vi "SeCrTs-Data queue.vi"(3 "error in":errorcluster) -> (7 "Data FIFO Ref":T1, 10 "error out":errorcluster)   [LabVIEW 2022 SP3]
uses:
  RT Controls/SeCrTs-Data FIFO.ctl
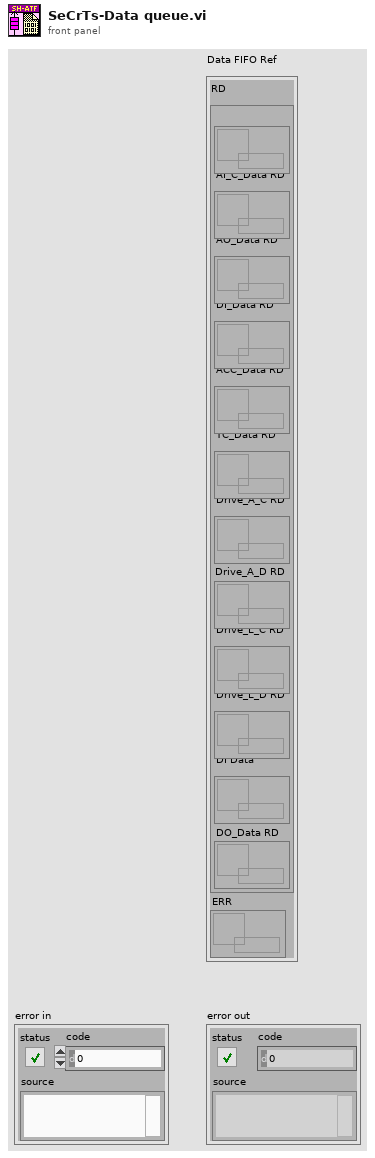
[diagram p1: front panel]
types:
  T1 = typedef "SeCrTs-Data FIFO.ctl" = cluster{"RD":cluster{"AI_V_Data RD":refnum<queue>, "AI_C_Data RD":refnum<queue>, "AO_Data RD":refnum<queue>, "DI_Data RD":refnum<queue>, "ACC_Data RD":refnum<queue>, "TC_Data RD":refnum<queue>, "Drive_A_C RD":refnum<queue>, "Drive_A_D RD":refnum<queue>, "Drive_L_C RD":refnum<queue>, "Drive_L_D RD":refnum<queue>, "DI Data":refnum<queue>, "DO_Data RD":refnum<queue>}, "ERR":refnum<queue>}
  T2 = cluster{"Error Code":string, "Error Source":string}
  T3 = cluster{"AI_V_Data RD":refnum<queue>, "AI_C_Data RD":refnum<queue>, "AO_Data RD":refnum<queue>, "DI_Data RD":refnum<queue>, "ACC_Data RD":refnum<queue>, "TC_Data RD":refnum<queue>, "Drive_A_C RD":refnum<queue>, "Drive_A_D RD":refnum<queue>, "Drive_L_C RD":refnum<queue>, "Drive_L_D RD":refnum<queue>, "DI Data":refnum<queue>, "DO_Data RD":refnum<queue>}
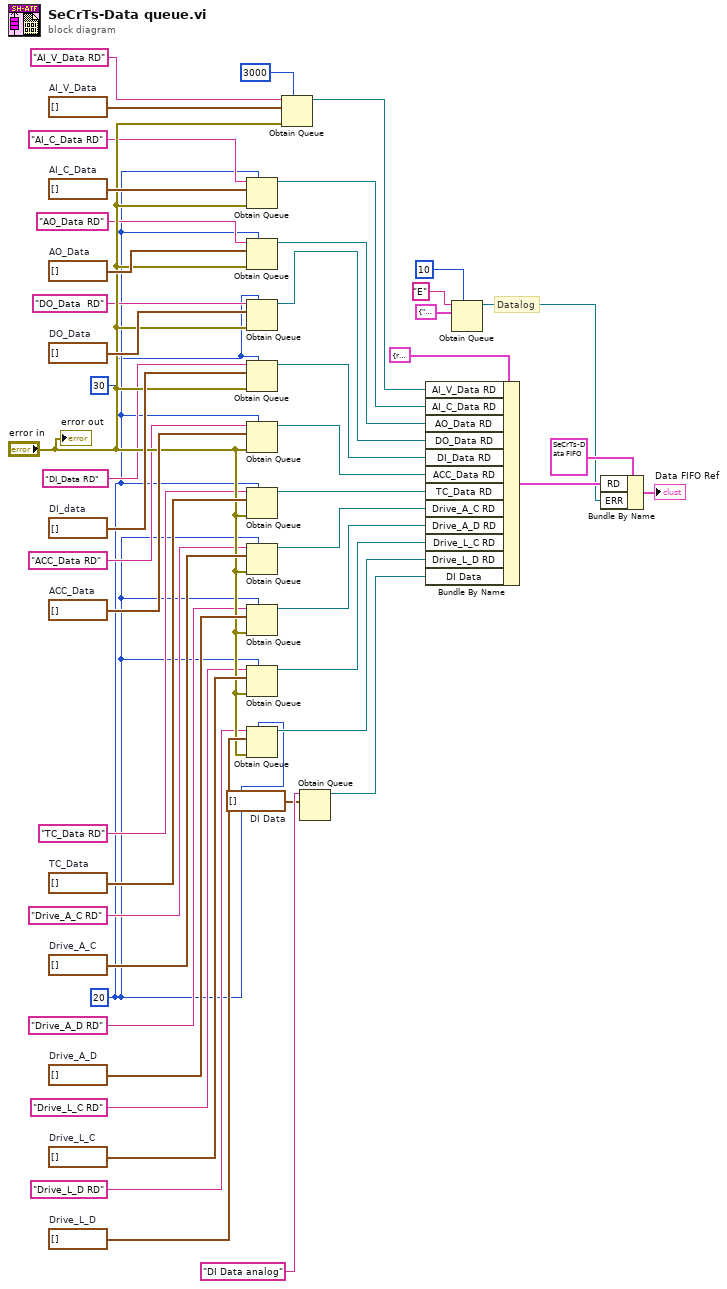
[diagram p0: block diagram]
diagram:
  w5 = 30 ("max queue size (-1, unlimited)")
  w10 = waveform(dbl)[] []  # DI Data
  w8 = 20 ("max queue size (-1, unlimited)")
  w48 = waveform(dbl)[] []  # AI_V_Data
  w38 = waveform(dbl)[] []  # Drive_L_D
  w39 = waveform(dbl)[] []  # Drive_L_C
  w40 = waveform(dbl)[] []  # Drive_A_D
  w41 = waveform(dbl)[] []  # Drive_A_C
  w42 = waveform(dbl)[] []  # TC_Data
  w43 = waveform(dbl)[] []  # ACC_Data
  w45 = digitalwaveform[] []  # DI_data
  w44 = waveform(dbl)[] []  # DO_Data
  w46 = waveform(dbl)[] []  # AO_Data
  w47 = waveform(dbl)[] []  # AI_C_Data
  # "Datalog"
  n1 = Obtain Queue(max queue size (-1, unlimited)=w8, name (unnamed)="AI_C_Data RD", element data type=w47, error in (no error)="error in") -> (queue out=w35:refnum<queue>)  [unwired: 1 in, 2 out]
  n2 = Obtain Queue(max queue size (-1, unlimited)=w8, name (unnamed)="AO_Data RD", element data type=w46, error in (no error)="error in") -> (queue out=w34:refnum<queue>)  [unwired: 1 in, 2 out]
  n3 = Obtain Queue(max queue size (-1, unlimited)=w5, name (unnamed)="DO_Data  RD", element data type=w44, error in (no error)="error in") -> (queue out=w33:refnum<queue>)  [unwired: 1 in, 2 out]
  n4 = Obtain Queue(max queue size (-1, unlimited)=w5, name (unnamed)="DI_Data RD", element data type=w45, error in (no error)="error in") -> (queue out=w32:refnum<queue>)  [unwired: 1 in, 2 out]
  n5 = Obtain Queue(max queue size (-1, unlimited)=w8, name (unnamed)="ACC_Data RD", element data type=w43, error in (no error)="error in") -> (queue out=w31:refnum<queue>)  [unwired: 1 in, 2 out]
  n6 = Obtain Queue(max queue size (-1, unlimited)=w8, name (unnamed)="TC_Data RD", element data type=w42, error in (no error)="error in") -> (queue out=w30:refnum<queue>)  [unwired: 1 in, 2 out]
  n7 = Obtain Queue(max queue size (-1, unlimited)=w8, name (unnamed)="Drive_A_C RD", element data type=w41, error in (no error)="error in") -> (queue out=w29:refnum<queue>)  [unwired: 1 in, 2 out]
  n8 = Obtain Queue(max queue size (-1, unlimited)=w8, name (unnamed)="Drive_A_D RD", element data type=w40, error in (no error)="error in") -> (queue out=w28:refnum<queue>)  [unwired: 1 in, 2 out]
  n9 = Obtain Queue(max queue size (-1, unlimited)=w8, name (unnamed)="Drive_L_C RD", element data type=w39, error in (no error)="error in") -> (queue out=w27:refnum<queue>)  [unwired: 1 in, 2 out]
  n10 = Obtain Queue(max queue size (-1, unlimited)=w8, name (unnamed)="Drive_L_D RD", element data type=w38, error in (no error)="error in") -> (queue out=w26:refnum<queue>)  [unwired: 1 in, 2 out]
  n11 = Obtain Queue(max queue size (-1, unlimited)=3000, name (unnamed)="AI_V_Data RD", element data type=w48, error in (no error)="error in") -> (queue out=w37:refnum<queue>)  [unwired: 1 in, 2 out]
  n12 = Obtain Queue(name (unnamed)="DI Data analog", element data type=w10) -> (queue out=w9:refnum<queue>)  [unwired: 3 in, 2 out]
  n13 = Bundle By Name(cluster=T3 {"AI_V_Data RD"=refnum, "AI_C_Data RD"=refnum, "AO_Data RD"=refnum, "DI_Data RD"=refnum, "ACC_Data RD"=refnum, "TC_Data RD"=refnum, "Drive_A_C RD"=refnum, "Drive_A_D RD"=refnum, "Drive_L_C RD"=refnum, "Drive_L_D RD"=refnum, "DI Data"=refnum, "DO_Data RD"=refnum}, "AI_V_Data RD"=w37, "AI_C_Data RD"=w35, "AO_Data RD"=w34, "DO_Data RD"=w33, "DI_Data RD"=w32, "ACC_Data RD"=w31, "TC_Data RD"=w30, "Drive_A_C RD"=w29, "Drive_A_D RD"=w28, "Drive_L_C RD"=w27, "Drive_L_D RD"=w26, "DI Data"=w9) -> (w6:T3)
  n14 = Obtain Queue(max queue size (-1, unlimited)=10, name (unnamed)="E", element data type=T2 {"Error Code"="", "Error Source"=""} ("element")) -> (queue out=w1:refnum<queue>)  [unwired: 2 in, 2 out]
  n15 = Bundle By Name(cluster=T1 {"RD"={"AI_V_Data RD"=refnum, "AI_C_Data RD"=refnum, "AO_Data RD"=refnum, "DI_Data RD"=refnum, "ACC_Data RD"=refnum, "TC_Data RD"=refnum, "Drive_A_C RD"=refnum, "Drive_A_D RD"=refnum, "Drive_L_C RD"=refnum, "Drive_L_D RD"=refnum, "DI Data"=refnum, "DO_Data RD"=refnum}, "ERR"=refnum} ("Data FIFO Ref"), "RD"=w6, "ERR"=w1) -> (→"Data FIFO Ref":T1)
  "error out" <- "error in"
